vi "GetPTZConfig.vi"(7 "HTTP_address":string, 8 "error in (no error)":errorcluster, 10 "Value":T2, 11 "Refnum in":T1) -> (0 "error out":errorcluster, 3 "headers":string)   [LabVIEW 2016]
uses:
  cgi_string.ctl
  <vilib>/httpClient/ClientHandle.ctl
  <vilib>/httpClient/LabVIEWHTTPClient.lvlib
panel:
  out "http:":string
  out "body":string
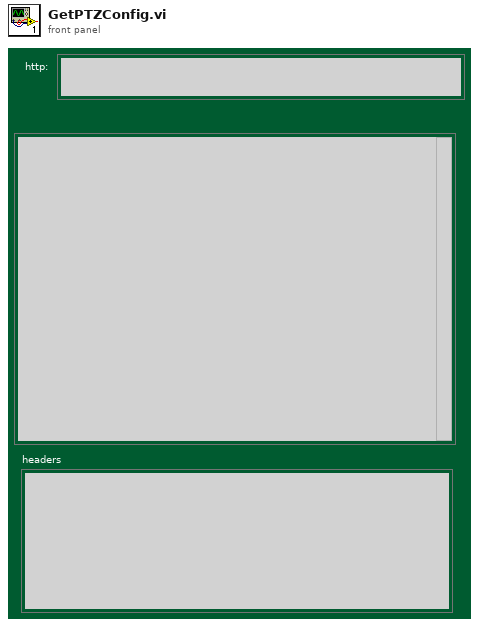
[diagram p1: front panel]
types:
  T1 = typedef "LabVIEWHTTPClient.lvlib/ClientHandle.ctl" = refnum<k1>
  T2 = typedef "cgi_string.ctl" = string
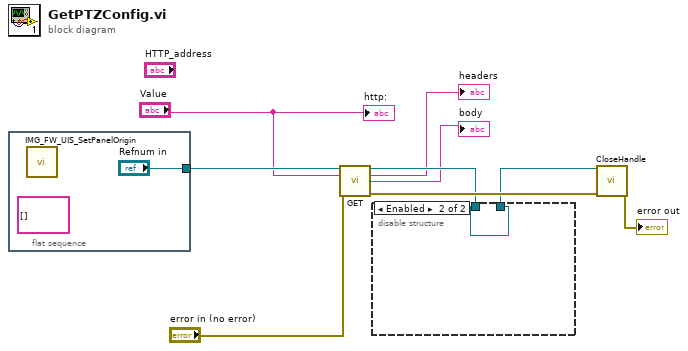
[diagram p0: block diagram]
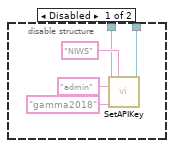
[diagram p2: hidden frame]
diagram:
  n1 = flat-sequence {
    tunnel: ["Refnum in"] -> w6
    frame #0 {
      (unwired) string[][] [] ("Table Control")
      n2 = call "IMG_FW_UIS_SetPanelOrigin.vi"() -> ()  [unwired: 11 in, 1 out]
    }
  }
  n3 = call <vilib>:"GET.vi"("client handle"=w6, "url"="Value", "error in (no error)"="error in (no error)") -> ("client handle out"=w5:T1, "headers"=→"headers":string, "body"=→"body":string, "error out"=w9:errorcluster)  [unwired: 9 in]
  n4 = disable-structure shown="Enabled" {
    disable-tunnel: w5 -> [w12 w16]
    disable-tunnel: [w11 w16] -> w4
    frame Disabled {
      n5 = call <vilib>:"SetAPIKey.vi"("client handle"=w12, "mode"="NIWS", "access id"="admin", "secret id"="gamma2018") -> ("client handle out"=w11:T1)  [unwired: 10 in, 1 out]
    }
    frame Enabled {
    }
  }
  n6 = call <vilib>:"CloseHandle.vi"("client handle"=w4, "error in (no error)"=w9) -> ("error out"=→"error out":errorcluster)  [unwired: 13 in]
  "http:" <- "Value"
